vi "Main.vi"() -> ()   [LabVIEW 2017]
doc: "The myRIO Project template acquires acceleration data from the onboard accelerometer and displays the changes of acceleration values in a waveform chart."
uses:
  <vilib>/myRIO/Common/Instrument Driver Framework/myRIO v1.0/Encoder/typedefs/Encoder Count Direction Enum.ctl
  Control 1.ctl
  <vilib>/myRIO/Instrument Drivers/Onboard IO/PWM/typedefs/PWM Reference.ctl
  <vilib>/myRIO/Common/Instrument Driver Framework/Utilities/typedefs/myRIO Generic Hardware Reference.ctl
  <vilib>/myRIO/Common/Instrument Driver Framework/Utilities/typedefs/Hardware Version Enum.ctl
  <vilib>/myRIO/Common/Instrument Driver Framework/Utilities/typedefs/myRIO v1.0 Reference.ctl
  <vilib>/myRIO/Common/Instrument Driver Framework/Utilities/typedefs/Generic FPGA Reference.ctl
  <vilib>/myRIO/Common/Instrument Driver Framework/myRIO v1.0/PWM/typedefs/PWM Channels Enum.ctl
  <vilib>/myRIO/Instrument Drivers/Onboard IO/PWM/typedefs/PWM Configuration.ctl
  <vilib>/userdefined/High Color/nirio_resource_hc.ctl
  <vilib>/myRIO/Common/Instrument Driver Framework/Utilities/vis/Is FPGA Ref Available.vi
  <vilib>/myRIO/Common/Instrument Driver Framework/myRIO v1.0/PWM/vis/myRIO v1.1 Open PWM.vi
  <vilib>/myRIO/Instrument Drivers/Onboard IO/PWM/vis/Set Duty Cycle and Frequency.vi
  <vilib>/myRIO/Common/Instrument Driver Framework/Utilities/vis/Validate Channels.vi
  <vilib>/myRIO/Common/Instrument Driver Framework/myRIO v1.0/PWM/vis/myRIO v1.0 Reserve PWM.vi
  <vilib>/myRIO/Common/Instrument Driver Framework/myRIO v1.0/UART/vis/myRIO v1.0 Close UART.vi
  <vilib>/myRIO/Common/Instrument Driver Framework/myRIO v1.0/PWM/vis/myRIO v1.0 Build MUX Configuration PWM.vi
  <vilib>/myRIO/Common/Instrument Driver Framework/myRIO v1.0/Resource Manager/vis/myRIO v1.0 Reserve Channel List.vi
  <vilib>/myRIO/Common/Instrument Driver Framework/myRIO v1.0/Resource Manager/vis/myRIO v1.0 Create Configuration List.vi
  <vilib>/myRIO/Common/Instrument Driver Framework/myRIO v1.0/Resource Manager/vis/myRIO v1.0 Reserve Channel.vi
  <vilib>/myRIO/Common/Instrument Driver Framework/myRIO v1.0/Resource Manager/vis/myRIO v1.0 Unreserve Channel.vi
  <vilib>/myRIO/Common/Instrument Driver Framework/myRIO v1.0/Resource Manager/vis/myRIO v1.0 Build Mutex Name.vi
  <vilib>/Utility/VariantDataType/GetNumericInfo.vi
  <vilib>/Utility/error.llb/Error Cluster From Error Code.vi
  <vilib>/myRIO/Common/Instrument Driver Framework/myRIO v1.0/myRIO v1.1 Open.vi
  <vilib>/myRIO/Common/Instrument Driver Framework/Utilities/vis/IO Manager.vi
  <vilib>/myRIO/Common/Instrument Driver Framework/Utilities/vis/Configuration Manager.vi
  <vilib>/myRIO/Common/Instrument Driver Framework/myRIO v1.0/Resource Manager/vis/myRIO v1.0 Configure IO.vi
  <vilib>/myRIO/Common/Instrument Driver Framework/myRIO v1.0/myRIO v1.0 Close.vi
  <vilib>/myRIO/Common/Instrument Driver Framework/myRIO v1.0/PWM/vis/myRIO v1.0 Write PWM.vi
  <vilib>/myRIO/Common/Instrument Driver Framework/Utilities/vis/FPGA Ref Manager.vi
  <vilib>/myRIO/Common/Instrument Driver Framework/myRIO v1.0/myRIO v1.0 Reset FPGA.vi
  <vilib>/myRIO/Common/Instrument Driver Framework/myRIO v1.0/IRQ/vis/myRIO v1.0 IRQ Info FGV.vi
  <vilib>/myRIO/Common/Instrument Driver Framework/myRIO v1.0/IRQ/vis/myRIO v1.0 Timer IRQ Info FGV.vi
  <vilib>/myRIO/Common/Instrument Driver Framework/myRIO v1.0/IRQ/vis/myRIO v1.0 ISR Agent.vi
  <vilib>/myRIO/Express VI/Onboard IO/PWM/PWM Express VI.xnode
  <vilib>/myRIO/Instrument Drivers/Onboard IO/PWM/vis/myRIO PWM Open.xnode
  <vilib>/myRIO/Instrument Drivers/Utilities/Utilities.lvlib
  <vilib>/myRIO/Instrument Drivers/Onboard IO/PWM/PWM.lvlib
panel:
  in  "Distance Target":T1
  in  "X Axis Motor Target":T2
  out "X Axis Motor Params":T3
  in  "Y Axis Motor Target":T4
  out "Y Axis Motor Params":T4
  in  "stop":bool
  out "Output String":string
  out "Encoder Output":T6
  out "Loop Iteration":i32
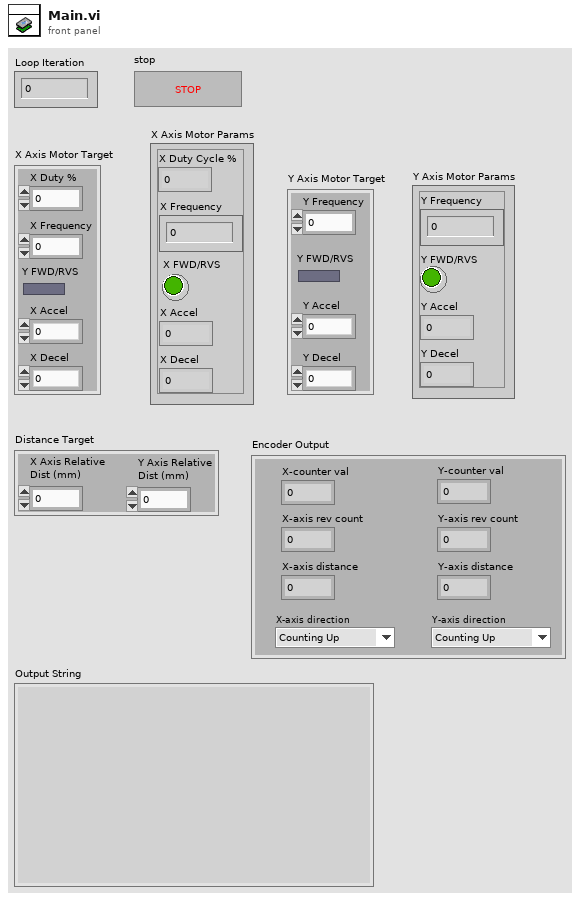
[diagram p1: front panel]
types:
  T1 = cluster{"X Axis Relative\nDist (mm)":dbl, "Y Axis Relative\nDist (mm)":dbl}
  T2 = cluster{"X Frequency":dbl, "Y FWD/RVS":bool, "X Accel":dbl, "X Decel":dbl, "X Duty %":dbl}
  T3 = cluster{"X Frequency":dbl, "X FWD/RVS":bool, "X Accel":dbl, "X Decel":dbl, "X Duty Cycle %":dbl}
  T4 = cluster{"Y Frequency":dbl, "Y FWD/RVS":bool, "Y Accel":dbl, "Y Decel":dbl}
  T5 = typedef "Encoder Count Direction Enum.ctl" = enum16{"Counting Up", "Counting Down"}
  T6 = cluster{"Y-axis rev count":dbl, "Y-axis distance":dbl, "X-axis rev count":dbl, "X-axis distance":dbl, "Y-axis direction":T5, "X-axis direction":T5, "X-counter val":i32, "Y-counter val":i32}
  T7 = typedef "Control 1.ctl" = enum8{"Stop & Reset", "Get Input", "Forwards", "Backwards"}
  T8 = cluster{dbl, "X-axis distance":dbl, "X Duty Cycle %":dbl, "X Frequency":dbl, "Y-axis distance":dbl, "Y Frequency":dbl, "X Accel":dbl, "X Decel":dbl, "Y Accel":dbl, "Y Decel":dbl}
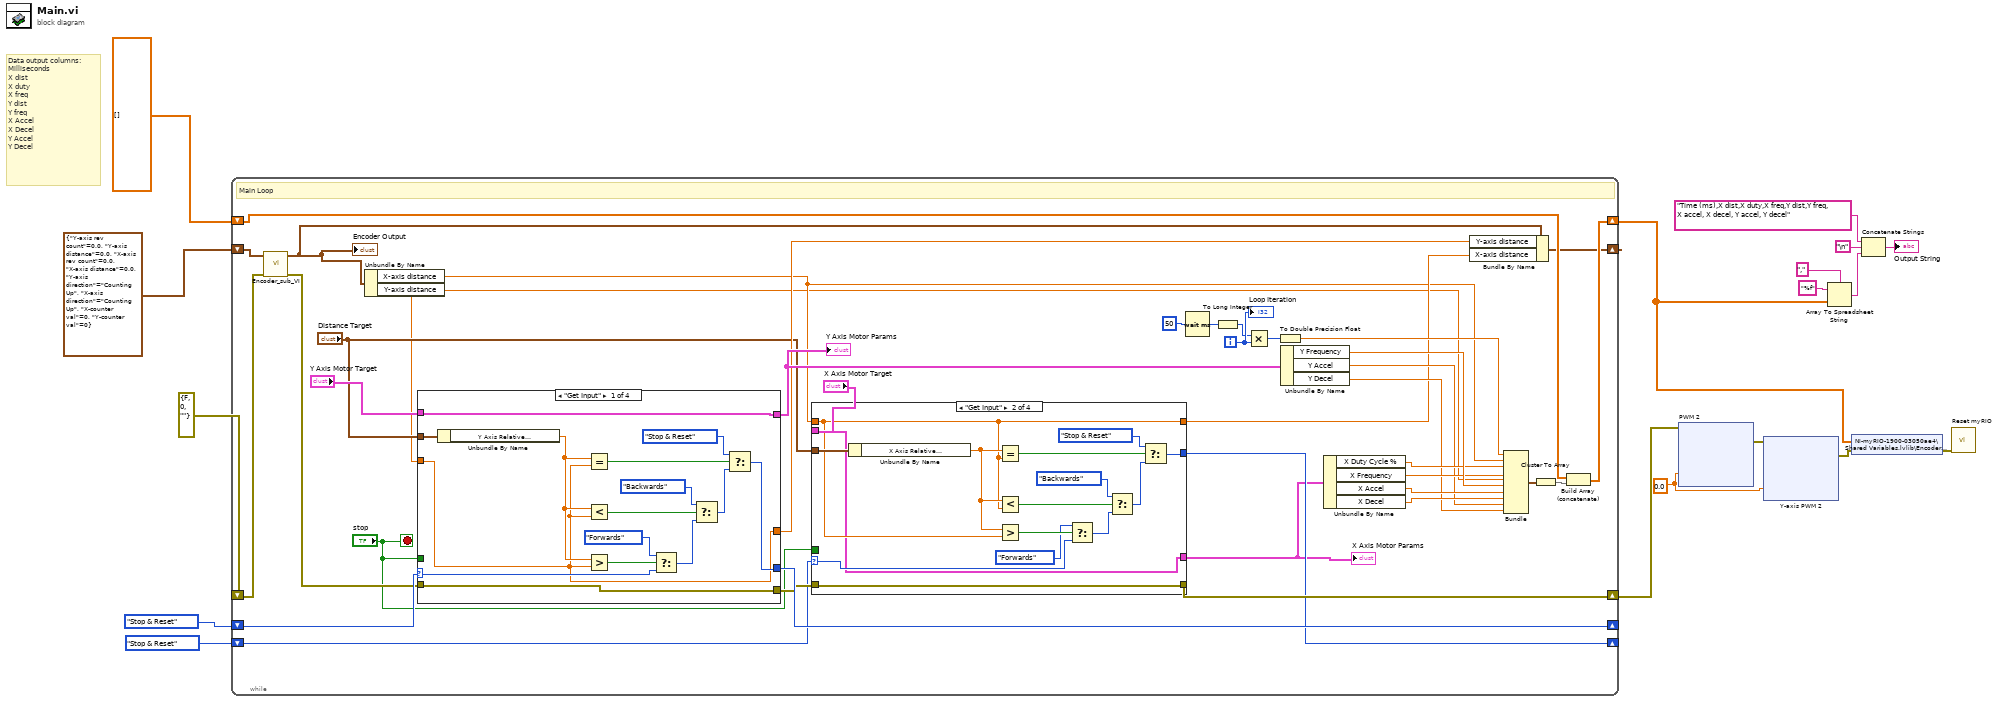
[diagram p0: block diagram]
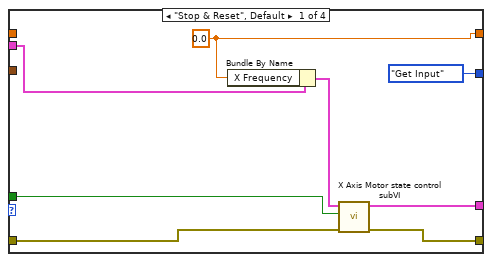
[diagram p2: hidden frame]
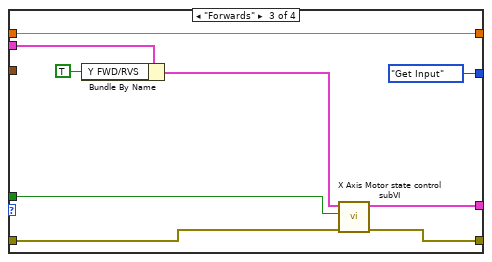
[diagram p3: hidden frame]
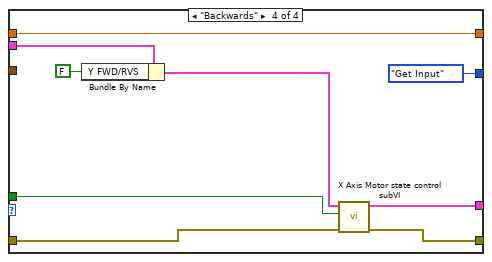
[diagram p4: hidden frame]
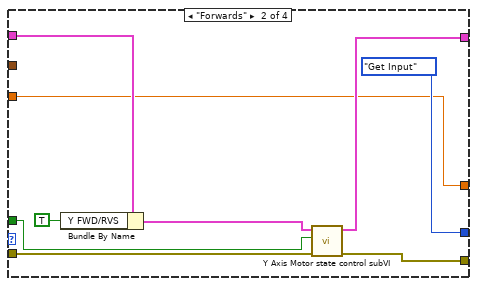
[diagram p5: hidden frame]
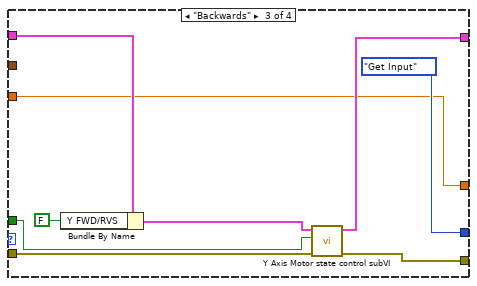
[diagram p6: hidden frame]
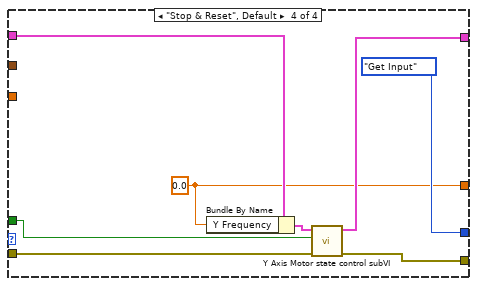
[diagram p7: hidden frame]
diagram:
  w4 = 0.0 ("Frequency [Hz]")
  # "Data output columns:\nMilliseconds\nX dist\nX duty\nX freq\nY dist\nY freq\nX Accel\nX Decel\nY Accel\nY Decel"
  n1 = while {
    shift-right: [w30] -> w17
    shift-left: errorcluster {"status"=FALSE, "code"=0, "source"=""} ("error in (no error)") -> [w55]
    shift-right: [w51] -> w7
    shift-left: dbl[][] [] -> [w46]
    shift-right: [w34] -> _
    shift-left: Control_1."Stop & Reset" -> [w35]
    shift-right: [w18] -> _
    shift-left: T6 {"Y-axis rev count"=0.0, "Y-axis distance"=0.0, "X-axis rev count"=0.0, "X-axis distance"=0.0, "Y-axis direction"=enum."Counting Up", "X-axis direction"=enum."Counting Up", "X-counter val"=0, "Y-counter val"=0} ("Encoder Input") -> [w37]
    shift-right: [w28] -> _
    shift-left: Control_1."Stop & Reset" -> [w29]
    i -> [w54]
    stop <- "stop" stop-if-true
    # "Main Loop"
    n2 = call "Encoder_sub_VI.vi"("error in (no error)"=w55, "Encoder Input"=w37) -> ("error out"=w32:errorcluster, "Encoder Output"=w22:T6)  [unwired: 8 in]
    "Encoder Output" <- w22
    n3 = Unbundle By Name(w22) -> ("X-axis distance"=w20:dbl, "Y-axis distance"=w19:dbl)
    n4 = case shown="\"Get Input\"" w35 {
      selector: w35 -> [w108 _ _ _]
      tunnel: "Y Axis Motor Target" -> [w99 w120 w127 w137]
      tunnel: [w102 Control_1."Get Input" Control_1."Get Input" Control_1."Get Input"] -> w34
      tunnel: "stop" -> [_ w117 w125 w133]
      tunnel: [w99 w116 w129 w135] -> w33
      tunnel: "Distance Target" -> [w111 _ _ _]
      tunnel: w32 -> [w98 w114 w123 w132]
      tunnel: [w98 w113 w122 w131] -> w31
      tunnel: [w97 w112 w121 w130] -> w24
      tunnel: w19 -> [w97 w112 w121 _]
      frame "Get Input" {
        n5 = Unbundle By Name(w111) -> ("Y Axis Relative\nDist (mm)"=w101:dbl)
        n6 = Equal?(x=w101, y=w97) -> (x = y?=w104:bool)
        n7 = Less?(x=w101, y=w97) -> (x < y?=w106:bool)
        n8 = Greater?(x=w101, y=w97) -> (0:w110:bool)
        n9 = Select(t=Control_1."Forwards", s=w110, f=w108) -> (s? t:f=w107:T7)
        n10 = Select(t=Control_1."Backwards", s=w106, f=w107) -> (s? t:f=w103:T7)
        n11 = Select(t=Control_1."Stop & Reset", s=w104, f=w103) -> (s? t:f=w102:T7)
      }
      frame "Forwards" {
        n12 = Bundle By Name(cluster=w120, "Y FWD/RVS"=TRUE) -> (w119:T4)
        n13 = call "Y Axis Motor state control subVI.vi"("error in (no error)"=w114, "stop"=w117, "Y Axis Motor Target"=w119) -> ("error out"=w113:errorcluster, "Y Axis Motor Params"=w116:T4)  [unwired: 7 in]
      }
      frame "Backwards" {
        n14 = Bundle By Name(cluster=w127, "Y FWD/RVS"=FALSE) -> (w126:T4)
        n15 = call "Y Axis Motor state control subVI.vi"("error in (no error)"=w123, "stop"=w125, "Y Axis Motor Target"=w126) -> ("error out"=w122:errorcluster, "Y Axis Motor Params"=w129:T4)  [unwired: 7 in]
      }
      frame "Stop & Reset", Default {
        w130 = 0.0 ("Y Frequency")
        n16 = Bundle By Name(cluster=w137, "Y Frequency"=w130) -> (w136:T4)
        n17 = call "Y Axis Motor state control subVI.vi"("error in (no error)"=w132, "stop"=w133, "Y Axis Motor Target"=w136) -> ("error out"=w131:errorcluster, "Y Axis Motor Params"=w135:T4)  [unwired: 7 in]
      }
    }
    "Y Axis Motor Params" <- w33
    n18 = case shown="\"Get Input\"" w29 {
      selector: w29 -> [_ w65 _ _]
      tunnel: w31 -> [w61 w78 w86 w94]
      tunnel: [w60 w78 w85 w93] -> w30
      tunnel: [Control_1."Get Input" w66 Control_1."Get Input" Control_1."Get Input"] -> w28
      tunnel: "X Axis Motor Target" -> [w59 w64 w82 w89]
      tunnel: [w62 w64 w83 w88] -> w26
      tunnel: "stop" -> [w57 _ w79 w91]
      tunnel: [w56 w70 w87 w96] -> w23
      tunnel: w20 -> [_ w70 w87 w96]
      tunnel: "Distance Target" -> [_ w71 _ _]
      frame "Stop & Reset", Default {
        w56 = 0.0 ("X Frequency")
        n19 = Bundle By Name(cluster=w59, "X Frequency"=w56) -> (w58:T2)
        n20 = call "X Axis Motor state control subVI.vi"("error in (no error)"=w61, "stop"=w57, "X Axis Motor Target"=w58) -> ("error out"=w60:errorcluster, "X Axis Motor Params"=w62:T3)  [unwired: 7 in]
      }
      frame "Get Input" {
        n21 = Unbundle By Name(w71) -> ("X Axis Relative\nDist (mm)"=w72:dbl)
        n22 = Equal?(x=w72, y=w70) -> (x = y?=w74:bool)
        n23 = Less?(x=w72, y=w70) -> (x < y?=w75:bool)
        n24 = Greater?(x=w72, y=w70) -> (0:w77:bool)
        n25 = Select(t=Control_1."Forwards", s=w77, f=w65) -> (s? t:f=w76:T7)
        n26 = Select(t=Control_1."Backwards", s=w75, f=w76) -> (s? t:f=w73:T7)
        n27 = Select(t=Control_1."Stop & Reset", s=w74, f=w73) -> (s? t:f=w66:T7)
      }
      frame "Forwards" {
        n28 = Bundle By Name(cluster=w82, "Y FWD/RVS"=TRUE) -> (w81:T2)
        n29 = call "X Axis Motor state control subVI.vi"("error in (no error)"=w86, "stop"=w79, "X Axis Motor Target"=w81) -> ("error out"=w85:errorcluster, "X Axis Motor Params"=w83:T3)  [unwired: 7 in]
      }
      frame "Backwards" {
        n30 = Bundle By Name(cluster=w89, "Y FWD/RVS"=FALSE) -> (w90:T2)
        n31 = call "X Axis Motor state control subVI.vi"("error in (no error)"=w94, "stop"=w91, "X Axis Motor Target"=w90) -> ("error out"=w93:errorcluster, "X Axis Motor Params"=w88:T3)  [unwired: 7 in]
      }
    }
    "X Axis Motor Params" <- w26
    n32 = Wait (ms)(milliseconds to wait=u32 50) -> (millisecond timer value=w44:u32)
    n33 = To Long Integer(number=w44) -> (32bit integer=w50:i32)
    n34 = Multiply(x=w50, y=w54) -> (x*y=w48:i32)
    n35 = To Double Precision Float(number=w48) -> (double precision float=w47:dbl)
    n36 = Unbundle By Name(w33) -> ("Y Frequency"=w45:dbl, "Y Accel"=w39:dbl, "Y Decel"=w38:dbl)
    n37 = Unbundle By Name(w26) -> ("X Duty Cycle %"=w43:dbl, "X Frequency"=w42:dbl, "X Accel"=w41:dbl, "X Decel"=w40:dbl)
    n38 = Bundle By Name(cluster=w22, "Y-axis distance"=w24, "X-axis distance"=w23) -> (w18:T6)
    n39 = Bundle(w47, "X-axis distance"=w20, "X Duty Cycle %"=w43, "X Frequency"=w42, "Y-axis distance"=w19, "Y Frequency"=w45, "X Accel"=w41, "X Decel"=w40, "Y Accel"=w39, "Y Decel"=w38) -> (w52:T8)  [unwired: 1 in]
    n40 = Cluster To Array(cluster=w52) -> (array=w53:dbl[])
    n41 = Build Array (concatenate)(w46, w53) -> (w51:dbl[][])
    "Loop Iteration" <- w54
  }
  n42 = xnode "PWM 2"("Frequency [Hz]"=w4, "error in (no error)"=w17) -> ("error out"=w6:errorcluster)
  n43 = xnode "Y-axis PWM 2"("Frequency [Hz]"=w4, "error in (no error)"=w6) -> ("error out"=w5:errorcluster)
  n44 = Array To Spreadsheet String(delimiter (Tab)=",", array=w7, 3:"%f" ("format string")) -> (spreadsheet string=w14:string)
  n45 = shared-variable "NI-myRIO-1900-03050ae4\\Shared Variables.lvlib\\Encoder Data"(w7, error in=w5) -> (error out=w8:errorcluster)
  n46 = Concatenate Strings("Time (ms),X dist,X duty,X freq,Y dist,Y freq, X accel, X decel, Y accel, Y decel", "\n", w14) -> (→"Output String":string)
  n47 = call <vilib>:"Reset myRIO.vi"("error in (no error)"=w8) -> ()  [unwired: 10 in, 1 out]
